vi "AM Remove Zero DC - 75.vi"(10 "Longest Temp Vector":dbl[](array[numeric]), 11 "Average SG":dbl[](array[numeric])) -> (3 "normalized SG Data":dbl[](array[numeric]))   [LabVIEW 2020, in "Test Driver.lvlib"]
uses:
  Test Driver.lvlib
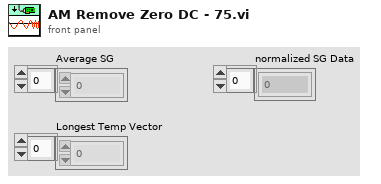
[diagram p1: front panel]
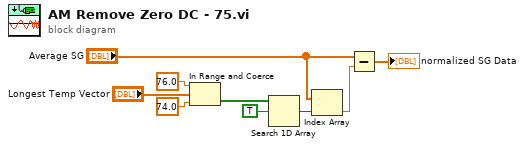
[diagram p0: block diagram]
diagram:
  n1 = In Range and Coerce(upper limit=76.0 ("R-square"), x="Longest Temp Vector", lower limit=74.0 ("R-square")) -> (In Range?=w3:bool[])  [unwired: 1 out]
  n2 = Search 1D Array(1D array=w3, element=TRUE) -> (index of element=w5:i32)  [unwired: 1 in]
  n3 = Index Array(array="Average SG", index=w5) -> (element=w6:dbl)
  n4 = Subtract(x="Average SG", y=w6) -> (x-y=→"normalized SG Data":dbl[])
